vi "Array_Remove empty columns (string).vi"(11 "Pockels Cal table":string[][](array[string])=[["Cal Wavelength", "", "", ""], ["820", "", "", ""], ["Prism 1:", "2039", "", ""], ["Prism 2:", "1953", "", ""], ["Laser power displayed (mW):", "3960", "", ""], ["Pockels bias:", "199", "", ""], ["Zoom:", "12", "", ""], ["Dwell time:", "0.4", "", ""], ["Cal subset indexes", "", "", ""], ["0", "15", "", ""], ["Cal data", "", "", ""], ["Pockels V", "No objective", "Nikon X", "Nikon 25X"], ["0", "0", "", "0"], ["0.1", "2.8", "", "1.96"], ["0.2", "9.8", "", "6.86"], ["0.3", "21.4", "", "14.98"], ["0.4", "37.1", "", "25.97"], ["0.5", "56.1", "", "39.27"], ["0.6", "77.7", "", "54.39"], ["0.7", "101", "", "70.7"], ["0.8", "125", "", "87.5"], ["0.9", "148", "", "103.6"], ["1", "169", "", "118.3"], ["1.1", "188", "", "131.6"], ["1.2", "204", "", "142.8"], ["1.3", "215", "", "150.5"], ["1.4", "222", "", "155.4"], ["1.5", "225", "", "157.5"], ["1.6", "222", "", "155.4"], ["1.7", "214", "", "149.8"], ["1.8", "202", "", "141.4"], ["1.9", "187", "", "130.9"], ["2", "152", "", "106.4"]]) -> (3 "Pockels Cal table (inc. header line)":string[][](array[string]))   [LabVIEW 2020]
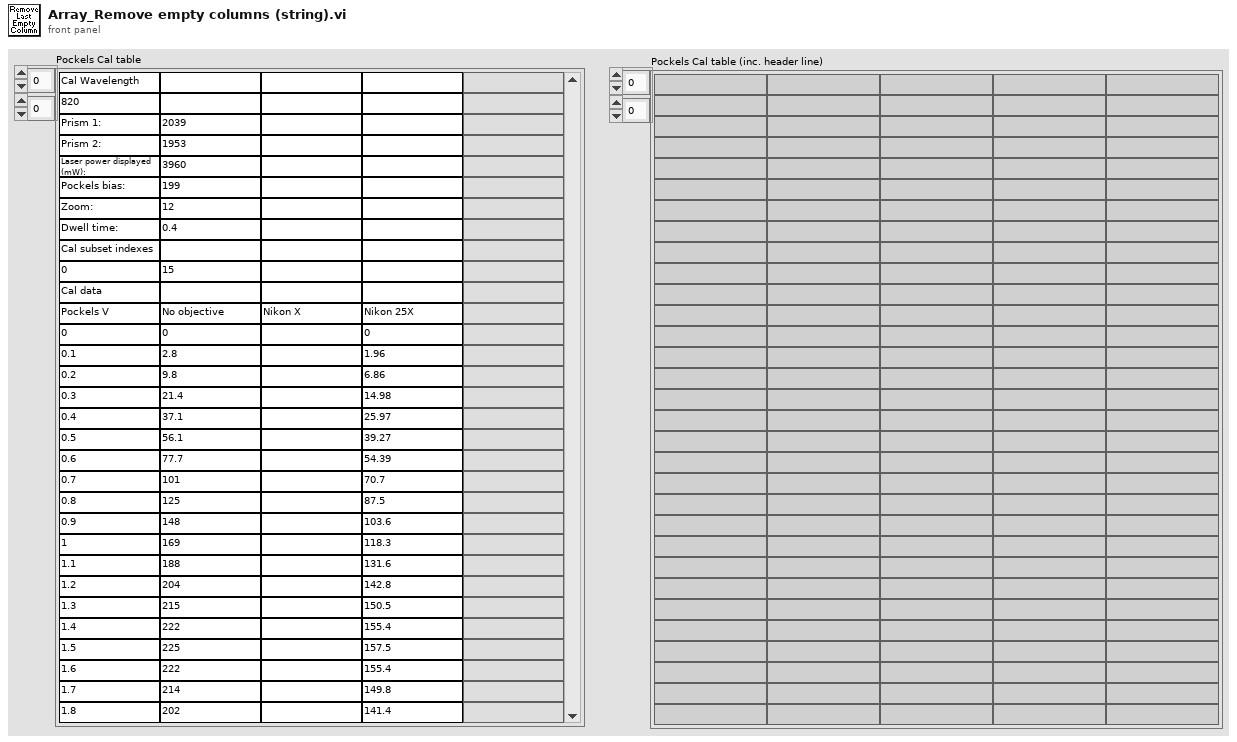
[diagram p1: front panel]
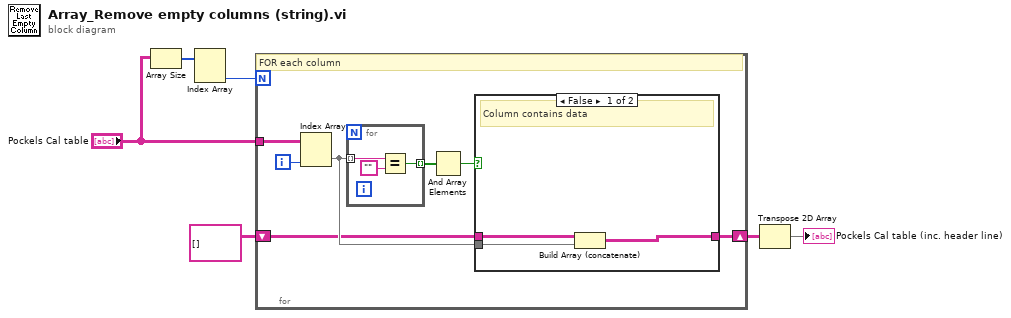
[diagram p0: block diagram]
diagram:
  n1 = Array Size(array="Pockels Cal table") -> (size(s)=w5:i32[])
  n2 = Index Array(array=w5) -> (element #2=w4:i32)  [unwired: 2 in, 1 out]
  n3 = for {
    N: w4 -> [_]
    tunnel: "Pockels Cal table" -> [w13]
    shift-right: [w7] -> w2
    shift-left: string[][] [] ("Pockels Cal table") -> [w8]
    i -> [w12]
    # "FOR each column"
    n4 = Index Array(array=w13, index (col)=w12) -> (element=w9:string[])  [unwired: 1 in]
    n5 = for {
      tunnel: w9 -> [w20] mode=indexing
      tunnel: [w18] -> w11 mode=indexing
      n6 = Equal?(x=w20, y="") -> (x = y?=w18:bool)
    }
    n7 = And Array Elements(Boolean array=w11) -> (logical AND=w10:bool)
    n8 = case shown="False" w10 {
      tunnel: w9 -> [w16 _]
      tunnel: w8 -> [w15 w17]
      tunnel: [w14 w17] -> w7
      frame False {
        # "Column contains data"
        n9 = Build Array (concatenate)(w15, w16) -> (w14:string[][])
      }
      frame True {
        # "Column is empty"
      }
    }
  }
  n10 = Transpose 2D Array(2D array=w2) -> (transposed array=→"Pockels Cal table (inc. header line)":string[][])
